vi "Shooter Code.vi"(10 "velocity_lower":dbl=1.0 format="%#_13g", 11 "velocity_upper":dbl=0.9 format="%#_13g") -> ()   [LabVIEW 2015]
panel:
  in  "lower limit":dbl=0.25
  in  "upper limit":dbl=0.25 format="%#_13g"
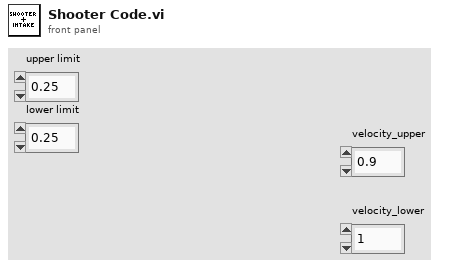
[diagram p1: front panel]
types:
  T1 = typedef "WPI_MotorControlDeviceRef.ctl" = cluster{"DeviceStatus":errorcluster, "Type":T2, "PWM":cluster{"PWM Channel":T3, "DeadBand":T4}, "CAN":cluster{"Device Number":u8, "Control Mode":T5, "Semaphore":T6, "Max Vout":dbl, "TalonSRX Control Mode":T7}, "Invert":bool}
  T2 = typedef "WPI_MotorControlType.ctl" = enum16{"PWM", "CAN", "CANTalonSRX"}
  T3 = typedef "FPGA_DIOPWMChannel.ctl" = enum8{"PWM 0", "PWM 1", "PWM 2", "PWM 3", "PWM 4", "PWM 5", "PWM 6", "PWM 7", "PWM 8", "PWM 9", "PWM MXP 0", "PWM MXP 1", "PWM MXP 2", "PWM MXP 3", "PWM MXP 4", "PWM MXP 5", "PWM MXP 6", "PWM MXP 7", "PWM MXP 8", "PWM MXP 9", "Invalid"}
  T4 = typedef "WPI_PWMDeadband.ctl" = cluster{"Name":string, "maxPositivePwm":i32, "minPositivePwm":i32, "centerPwm":i32, "maxNegativePwm":i32, "minNegativePwm":i32, "angularRange":u16}
  T5 = typedef "WPI_CANJaguar_ControlMode.ctl" = enum8{"Percent VBus", "Current", "Speed", "Position", "Voltage"}
  T6 = typedef "Semaphore RefNum" = refnum<k1>
  T7 = typedef "WPI_CANTalonSRX_APIControlMode.ctl" = enum8{"Percent VBus", "Speed", "Position", "Slave", "Unchanged / Invalid", "Voltage Compensation", "Current", "Motion Profile"}
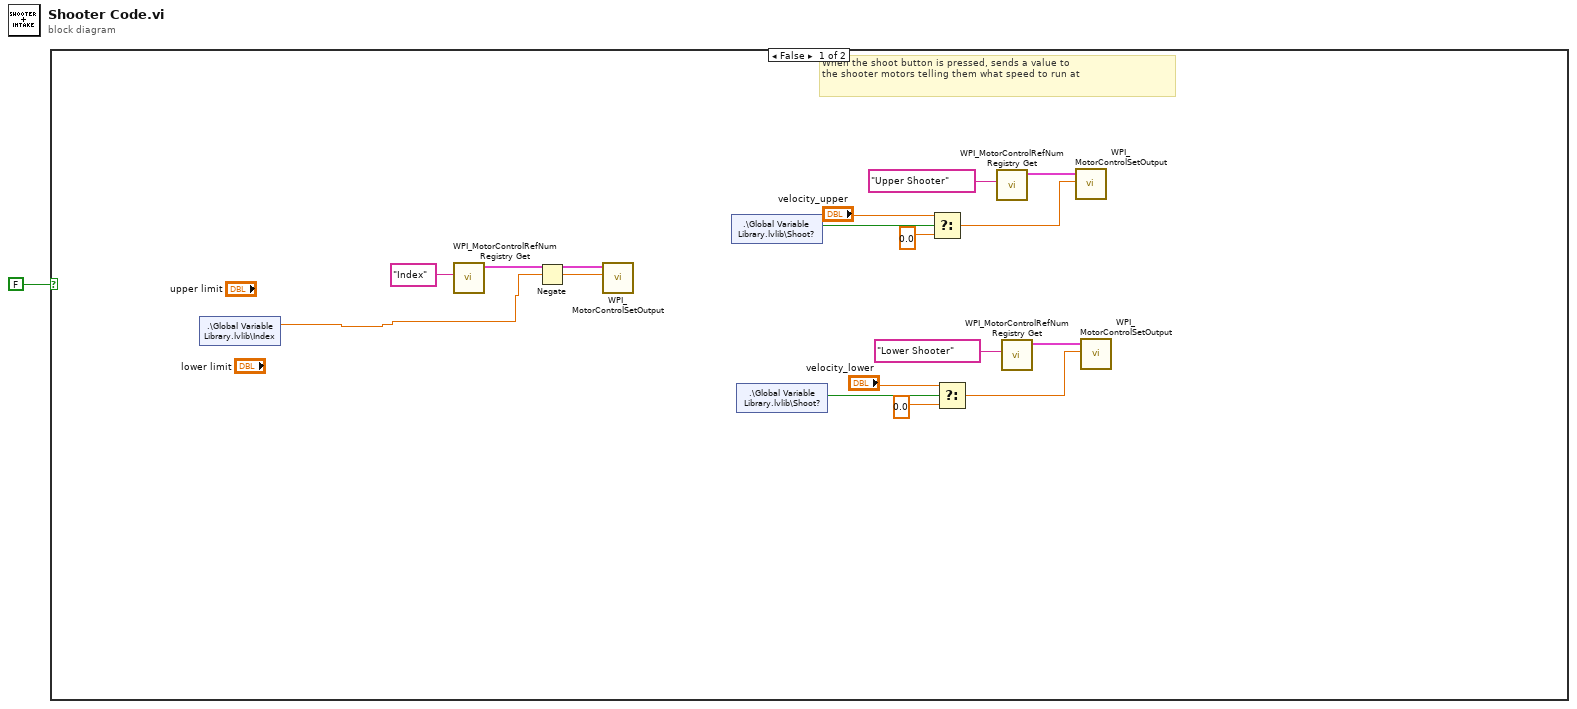
[diagram p0: block diagram]
diagram:
  n1 = case shown="False" FALSE {
    frame False {
      # "When the shoot button is pressed, sends a value to \nthe shooter motors telling them what speed to run at"
      n2 = shared-variable ".\\Global Variable Library.lvlib\\Index"() -> (w2:dbl)  [unwired: 1 in, 1 out]
      n3 = call <vilib>:"WPI_MotorControlRefNum Registry Get.vi"("refnum name"="Index") -> ("MotorControlDevRef"=w5:T1)  [unwired: 9 in, 1 out]
      n4 = Negate(x=w2) -> (-x=w3:dbl)
      n5 = call <vilib>:"WPI_MotorControlSetOutput.vi"("Output"=w3, "MotorControlDevRef"=w5) -> ()  [unwired: 7 in, 3 out]
      n6 = shared-variable ".\\Global Variable Library.lvlib\\Shoot?"() -> (w14:bool)  [unwired: 1 in, 1 out]
      n7 = shared-variable ".\\Global Variable Library.lvlib\\Shoot?"() -> (w9:bool)  [unwired: 1 in, 1 out]
      n8 = Select(t="velocity_upper", s=w14, f=0.0) -> (s? t:f=w17:dbl)
      n9 = Select(t="velocity_lower", s=w9, f=0.0 ("f 2")) -> (s? t:f=w6:dbl)
      n10 = call <vilib>:"WPI_MotorControlRefNum Registry Get.vi"("refnum name"="Upper Shooter") -> ("MotorControlDevRef"=w12:T1)  [unwired: 9 in, 1 out]
      n11 = call <vilib>:"WPI_MotorControlRefNum Registry Get.vi"("refnum name"="Lower Shooter") -> ("MotorControlDevRef"=w11:T1)  [unwired: 9 in, 1 out]
      n12 = call <vilib>:"WPI_MotorControlSetOutput.vi"("Output"=w17, "MotorControlDevRef"=w12) -> ()  [unwired: 7 in, 3 out]
      n13 = call <vilib>:"WPI_MotorControlSetOutput.vi"("Output"=w6, "MotorControlDevRef"=w11) -> ()  [unwired: 7 in, 3 out]
    }
    frame True {
    }
  }
